vi "fodase.vi"() -> ()   [LabVIEW 2013]
uses:
  <vilib>/Instr/_visa.llb/VISA Configure Serial Port (Instr).vi
panel:
  out "3":i32(graph)
  out "2":i32(graph)
  out "1":i32(graph)
  out "0":i32(graph)
  in  "stop":bool
  out "time":u32[](graph)
  out "cell":u8[](array[numeric])
  out "output_int16":i32[](array[numeric])
  out "data":u8[](array[numeric])
  in  "serial_port":refnum<visa-resource-name> caption="Porta Serial"
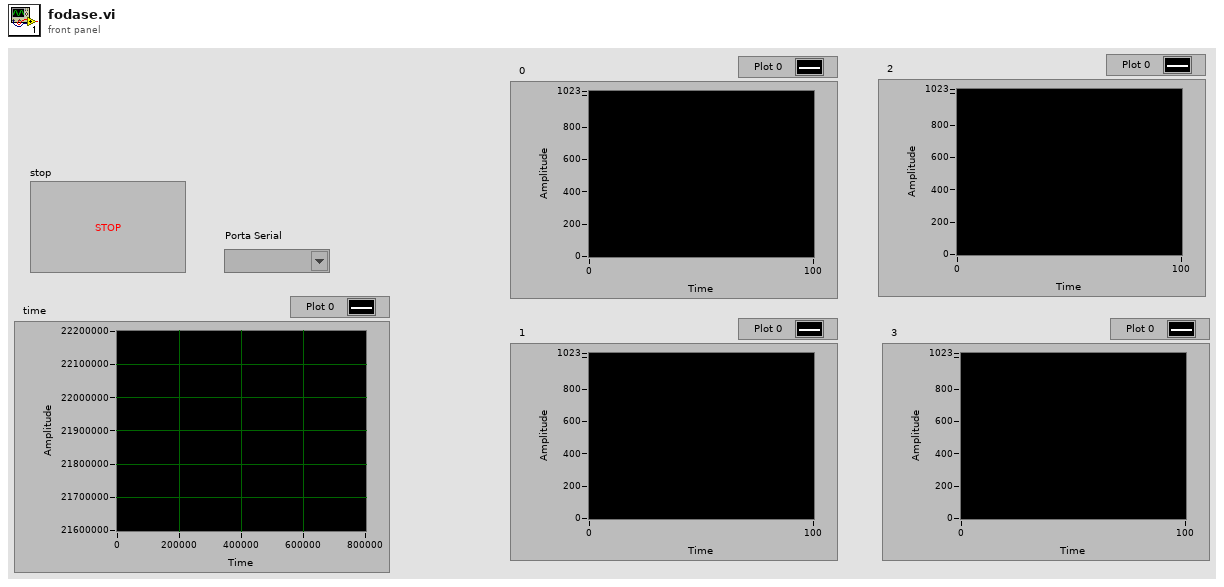
[diagram p1: front panel]
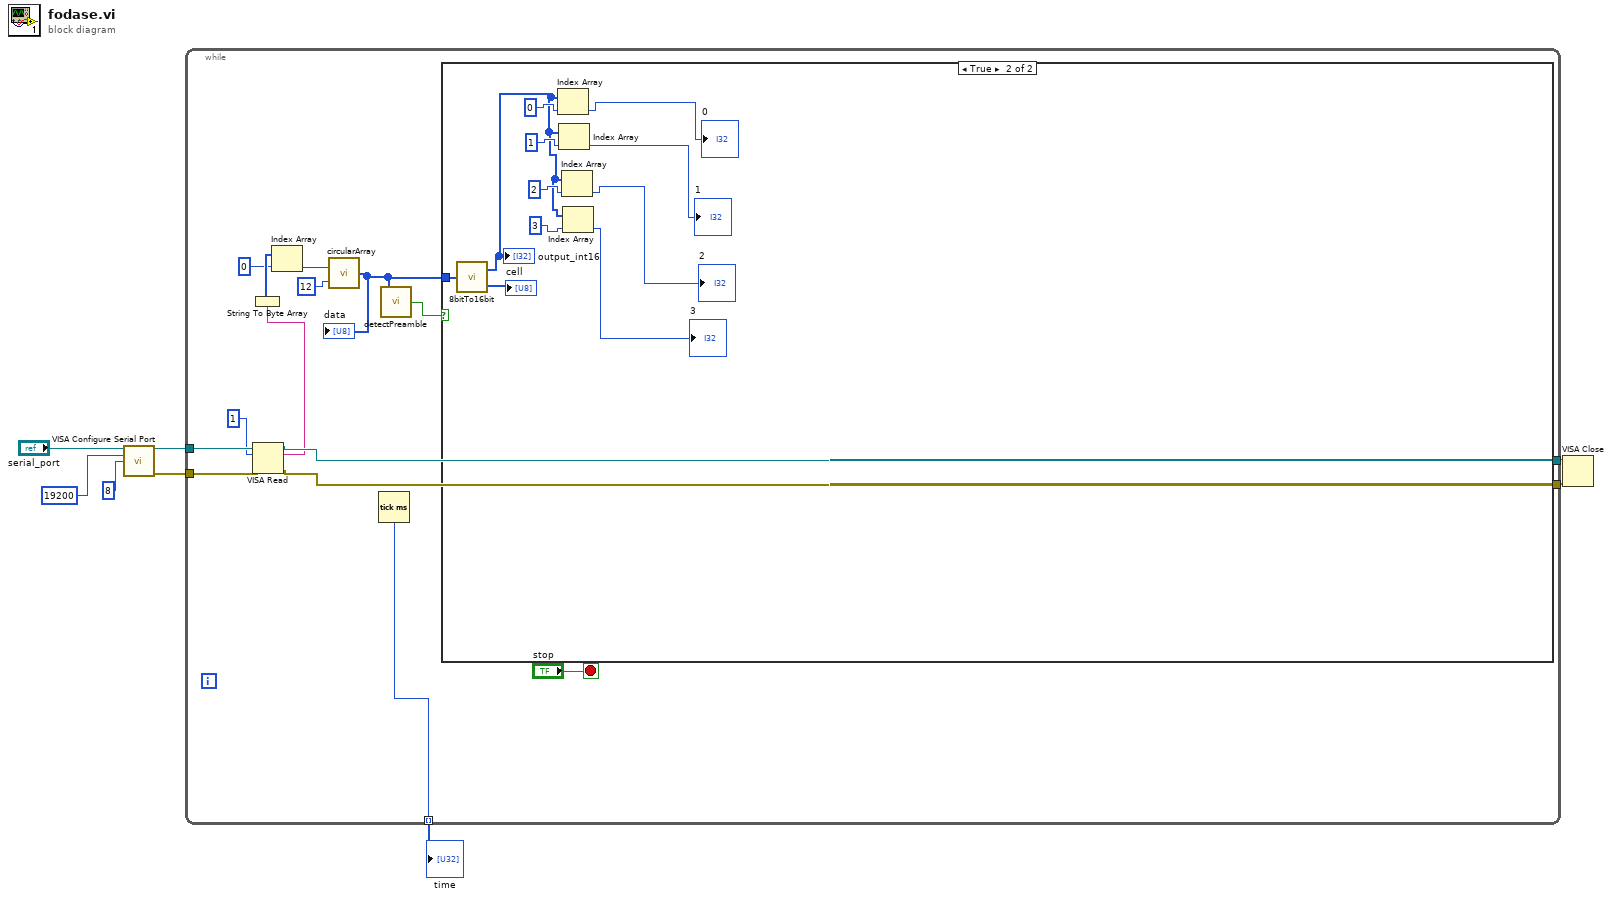
[diagram p0: block diagram]
diagram:
  n1 = call-poly "VISA Configure Serial Port"("VISA resource name"="serial_port", "baud rate (9600)"=u32 19200, "data bits (8)"=u16 8) -> ("VISA resource name out"=w5:refnum<visa-resource-name>, "error out"=w4:errorcluster)  [unwired: 11 in]
  n2 = while {
    tunnel: w5 -> [w22]
    tunnel: w4 -> [w21]
    tunnel: [w19] -> w2
    tunnel: [w20] -> w3
    tunnel: [w10] -> w1 mode=indexing
    stop <- "stop" stop-if-true
    n3 = VISA Read(VISA resource name=w22, byte count=1, error in (no error)=w21) -> (VISA resource name out=w20:refnum<visa-resource-name>, read buffer=w14:string, error out=w19:errorcluster)  [unwired: 1 out]
    n4 = String To Byte Array(string=w14) -> (unsigned byte array=w17:u8[])
    n5 = Index Array(array=w17, index=0) -> (element=w11:u8)
    n6 = call "circularArray.vi"("max-size"=u8 12, "element"=w11) -> ("dataout"=w12:u8[])
    "data" <- w12
    n7 = Tick Count (ms)() -> (millisecond timer value=w10:u32)
    n8 = call "detectPreamble.vi"("data-in"=w12) -> ("detected"=w9:bool)
    n9 = case shown="True" w9 {
      tunnel: w12 -> [_ w32]
      frame False {
      }
      frame True {
        n10 = call "8bitTo16bit.vi"("input_byte"=w32) -> ("output_int16"=w27:i32[], "cell"=→"cell":u8[])
        "output_int16" <- w27
        n11 = Index Array(array=w27, index=0) -> (element=→"0":i32)
        n12 = Index Array(array=w27, index=1) -> (element=→"1":i32)
        n13 = Index Array(array=w27, index=2) -> (element=→"2":i32)
        n14 = Index Array(array=w27, index=3) -> (element=→"3":i32)
      }
    }
  }
  "time" <- w1
  n15 = VISA Close(VISA resource name=w3, error in (no error)=w2) -> ()  [unwired: 1 out]
